vi "StringifiedData.vi"(8 "error in (no error)":errorcluster, 11 "ErrorMsg in":refnum<class "ErrorMsg.lvclass">) -> (0 "error out":errorcluster, 2 "Stringified Data":string, 3 "ErrorMsg out":refnum<class "ErrorMsg.lvclass">)   [LabVIEW 2017, in "LapDog.Messaging.v3.lvlib" / "ErrorMsg.lvclass"]
doc: "This VI is used for the message probe. Child classes may override it and provide the message data in string format or a short string describing the data the message contains. This string will be displayed in the probe window."
uses:
  ErrorMsg.lvclass
  ErrorMsg.lvclass/ErrorMsg.ctl
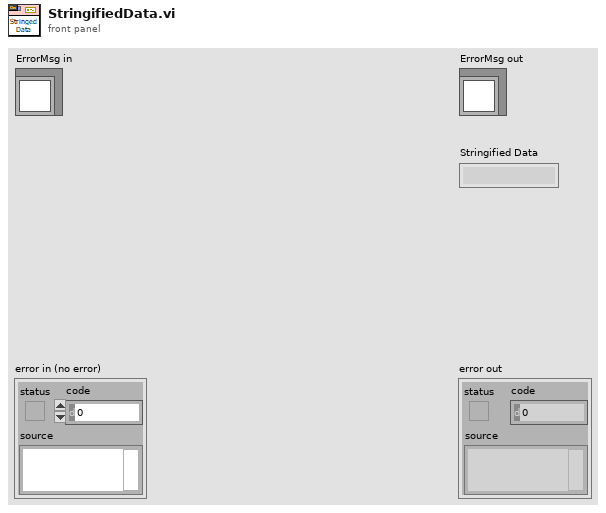
[diagram p1: front panel]
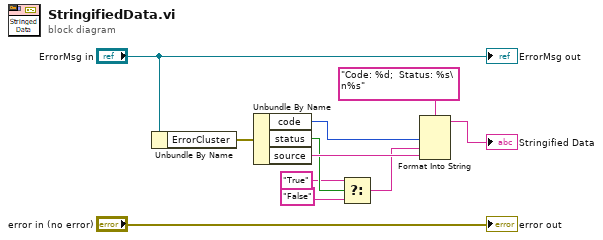
[diagram p0: block diagram]
diagram:
  n1 = Unbundle By Name("ErrorMsg in") -> ("ErrorCluster"=w9:errorcluster)
  n2 = Unbundle By Name(w9) -> ("code"=w7:i32, "status"=w4:bool, "source"=w8:string)
  n3 = Select(t="True", s=w4, f="False") -> (s? t:f=w1:string)
  n4 = Format Into String(format string="Code: %d;  Status: %s\n%s", w7, w1, w8) -> (resulting string=→"Stringified Data":string)  [unwired: 2 in, 1 out]
  "error out" <- "error in (no error)"
  "ErrorMsg out" <- "ErrorMsg in"
